vi "PM5000_Power_Metering_HMI.vi"(8 "error in":errorcluster, 11 "Network Path":string="172.22.26.202") -> (0 "error out":errorcluster, 1 "Power_array":sgl[](array[numeric]), 2 "Power Meter Out":T1, 3 "Network Path out":string="192.168.169.1")   [LabVIEW 2018]
doc: "Lee la tabla de memoria RealTime_VIF_Power del equipo PowerMonitor 5000, ademas filtra y ordena las variables de interez de la tabla de memoria.\n\nLee las siguientes variables de la tabla RealTime_VIF_Power:\n\n*V1_V2_Volts\n*V2_V3_Volts\n*V3_V1_Volts\n*I1_Amps\n*I2_Amps\n*I3_Amps\n*Frequency_Hz\n*Total_kW\n*Total_kVAR\n*Total_kVA\n*Total_True_PF\n*Total_Disp_PF"
uses:
  <vilib>/ethernetip/ethernetip.llb/EthernetIP SLC500 Read Float.vi
  <vilib>/ethernetip/ethernetip.lvlib
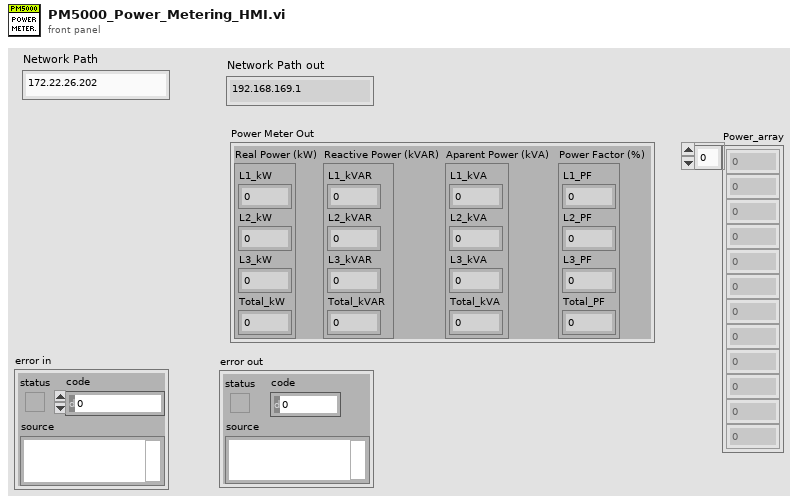
[diagram p1: front panel]
types:
  T1 = cluster{"Real Power (kW)":cluster{"L1_kW":sgl, "L2_kW":sgl, "L3_kW":sgl, "Total_kW":sgl}, "Reactive Power (kVAR)":cluster{"L1_kVAR":sgl, "L2_kVAR":sgl, "L3_kVAR":sgl, "Total_kVAR":sgl}, "Aparent Power (kVA)":cluster{"L1_kVA":sgl, "L2_kVA":sgl, "L3_kVA":sgl, "Total_kVA":sgl}, "Power Factor (%)":cluster{"L1_PF":sgl, "L2_PF":sgl, "L3_PF":sgl, "Total_PF":sgl}}
  T2 = cluster{"L1_PF":sgl, "L2_PF":sgl, "L3_PF":sgl, "Total_PF":sgl}
  T3 = cluster{"L1_kVA":sgl, "L2_kVA":sgl, "L3_kVA":sgl, "Total_kVA":sgl}
  T4 = cluster{"L1_kVAR":sgl, "L2_kVAR":sgl, "L3_kVAR":sgl, "Total_kVAR":sgl}
  T5 = cluster{"L1_kW":sgl, "L2_kW":sgl, "L3_kW":sgl, "Total_kW":sgl}
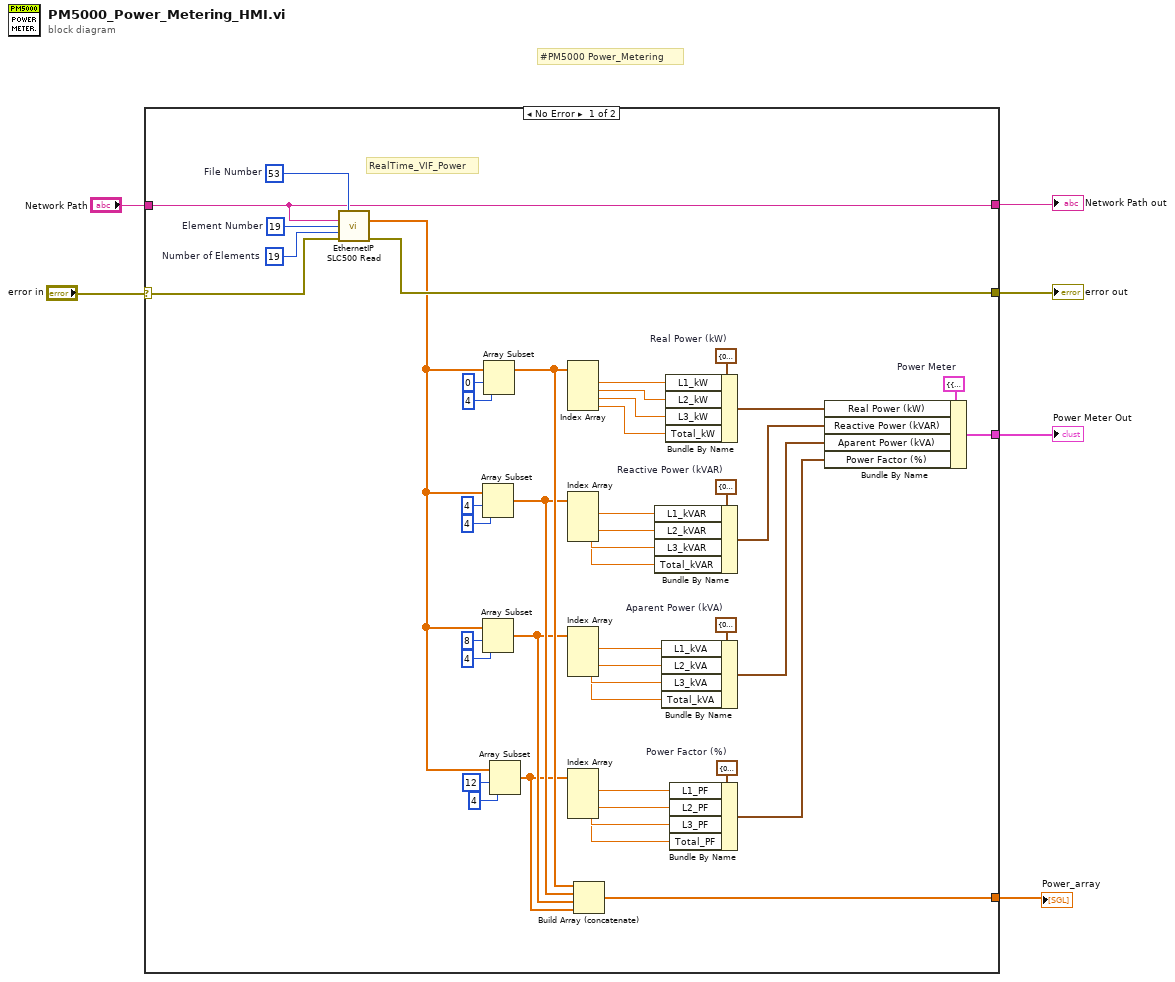
[diagram p0: block diagram]
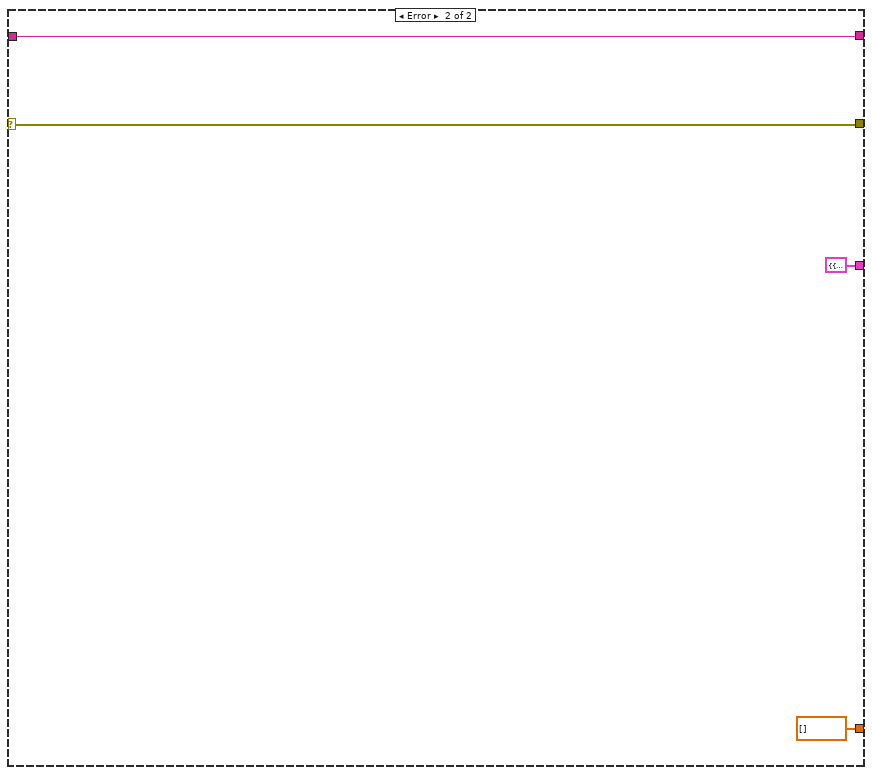
[diagram p2: hidden frame]
diagram:
  # "#PM5000 Power_Metering"
  n1 = case shown="No Error" "error in" {
    selector: "error in" -> [w13 w56]
    tunnel: [w52 w56] -> w6
    tunnel: [w8 w54] -> w5
    tunnel: [w14 T1 {"Real Power (kW)"={"L1_kW"=0.0, "L2_kW"=0.0, "L3_kW"=0.0, "Total_kW"=0.0}, "Reactive Power (kVAR)"={"L1_kVAR"=0.0, "L2_kVAR"=0.0, "L3_kVAR"=0.0, "Total_kVAR"=0.0}, "Aparent Power (kVA)"={"L1_kVA"=0.0, "L2_kVA"=0.0, "L3_kVA"=0.0, "Total_kVA"=0.0}, "Power Factor (%)"={"L1_PF"=0.0, "L2_PF"=0.0, "L3_PF"=0.0, "Total_PF"=0.0}} ("Power Meter")] -> w4
    tunnel: "Network Path" -> [w8 w54]
    tunnel: [w7 sgl[] []] -> w1
    frame No Error {
      w19 = T1 {"Real Power (kW)"={"L1_kW"=-0.009145112, "L2_kW"=-0.0037322815, "L3_kW"=-0.019452685, "Total_kW"=-0.03233008}, "Reactive Power (kVAR)"={"L1_kVAR"=-0.01587091, "L2_kVAR"=-0.0369946, "L3_kVAR"=-0.038295496, "Total_kVAR"=-0.091161005}, "Aparent Power (kVA)"={"L1_kVA"=0.018485848, "L2_kVA"=0.037469197, "L3_kVA"=0.04338286, "Total_kVA"=0.099337906}, "Power Factor (%)"={"L1_PF"=49.470882, "L2_PF"=9.960934, "L3_PF"=44.839565, "Total_PF"=32.545567}}  # Power Meter
      w41 = T2 {"L1_PF"=0.0, "L2_PF"=0.0, "L3_PF"=0.0, "Total_PF"=0.0}  # Power Factor (%)
      w42 = T3 {"L1_kVA"=0.0, "L2_kVA"=0.0, "L3_kVA"=0.0, "Total_kVA"=0.0}  # Aparent Power (kVA)
      w43 = T4 {"L1_kVAR"=0.0, "L2_kVAR"=0.0, "L3_kVAR"=0.0, "Total_kVAR"=0.0}  # Reactive Power (kVAR)
      w48 = T5 {"L1_kW"=0.0, "L2_kW"=0.0, "L3_kW"=0.0, "Total_kW"=0.0}  # Real Power (kW)
      w49 = u32 19  # Number of Elements
      w51 = u16 53  # File Number
      w50 = u16 19  # Element Number
      # "RealTime_VIF_Power"
      n2 = call-poly <vilib>:"EthernetIP SLC500 Read.vi"("File Number"=w51, "Network Path"=w8, "Element Number"=w50, "Number of Elements"=w49, "error in"=w13) -> ("Data"=w32:sgl[], "error out"=w52:errorcluster)  [unwired: 8 in, 1 out]
      n3 = Array Subset(array=w32, index=4, length=4) -> (w11:sgl[])
      n4 = Array Subset(array=w32, index=8, length=4) -> (w10:sgl[])
      n5 = Array Subset(array=w32, index=0, length=4) -> (w12:sgl[])
      n6 = Array Subset(array=w32, index=12, length=4) -> (w9:sgl[])
      n7 = Index Array(array=w12) -> (element #1=w47:sgl, element #2=w46:sgl, element #3=w45:sgl, element #4=w44:sgl)  [unwired: 4 in]
      n8 = Index Array(array=w11) -> (element #1=w31:sgl, element #2=w30:sgl, element #3=w29:sgl, element #4=w28:sgl)  [unwired: 4 in]
      n9 = Index Array(array=w10) -> (element #1=w27:sgl, element #2=w26:sgl, element #3=w25:sgl, element #4=w24:sgl)  [unwired: 4 in]
      n10 = Index Array(array=w9) -> (element #1=w23:sgl, element #2=w22:sgl, element #3=w21:sgl, element #4=w20:sgl)  [unwired: 4 in]
      n11 = Build Array (concatenate)(w12, w11, w10, w9) -> (w7:sgl[])
      n12 = Bundle By Name(cluster=w43, "L1_kVAR"=w31, "L2_kVAR"=w30, "L3_kVAR"=w29, "Total_kVAR"=w28) -> (w17:T4)
      n13 = Bundle By Name(cluster=w42, "L1_kVA"=w27, "L2_kVA"=w26, "L3_kVA"=w25, "Total_kVA"=w24) -> (w16:T3)
      n14 = Bundle By Name(cluster=w48, "L1_kW"=w47, "L2_kW"=w46, "L3_kW"=w45, "Total_kW"=w44) -> (w18:T5)
      n15 = Bundle By Name(cluster=w41, "L1_PF"=w23, "L2_PF"=w22, "L3_PF"=w21, "Total_PF"=w20) -> (w15:T2)
      n16 = Bundle By Name(cluster=w19, "Real Power (kW)"=w18, "Reactive Power (kVAR)"=w17, "Aparent Power (kVA)"=w16, "Power Factor (%)"=w15) -> (w14:T1)
    }
    frame Error {
    }
  }
  "error out" <- w6
  "Network Path out" <- w5
  "Power Meter Out" <- w4
  "Power_array" <- w1
